vi "Event_Unregister.vi"(1 "error in":errorcluster, 2 "Event Callback":refnum<k27>, 3 "DeviceStateChangedEvent":refnum<user-event>, 4 "Event Registration Refnum":refnum<event-registration>) -> (0 "error out":errorcluster)   [LabVIEW 2009]
uses:
  C:/Samples/LabVIEW/UseEventHandling/LabVIEW 2009/UsbDllWrap.dll
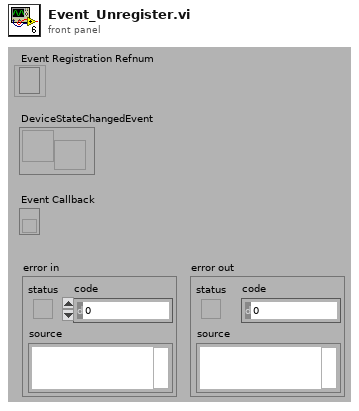
[diagram p1: front panel]
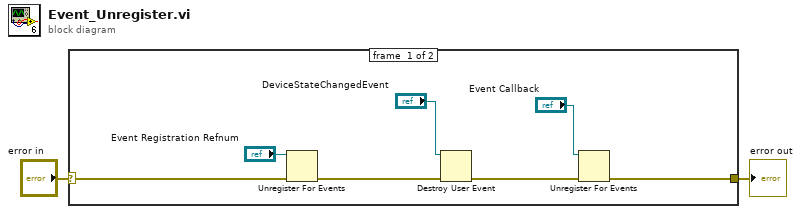
[diagram p0: block diagram]
diagram:
  n1 = case shown="No Error" "error in" {
    selector: "error in" -> [w5 w10]
    tunnel: [w9 w10] -> w2
    frame #0 {
      n2 = Unregister For Events(event registration refnum="Event Registration Refnum", error in=w5) -> (error out=w6:errorcluster)
      n3 = Destroy User Event(user event="DeviceStateChangedEvent", error in=w6) -> (error out=w7:errorcluster)
      n4 = Unregister For Events(event registration refnum="Event Callback", error in=w7) -> (error out=w9:errorcluster)
    }
    frame #1 {
    }
  }
  "error out" <- w2
